vi "LCD_Main Function.vi"(7 "Number of Matches Requested":i32, 8 "error in (no error)":errorcluster, 10 "ROI Descriptor":T3, 11 "Refnum in":T1) -> (0 "error out":errorcluster, 1 "Output value":dbl, 2 "ROI":T2={"Global Rectangle"=[], "Contours"=[{"Contour Type"=0, "ROI Type"=0, "Points"=[27, 55, 147, 27]}]}, 3 "Refnum out":T1)   [LabVIEW 2015]
uses:
  <vilib>/vision/Image Controls.llb/IMAQ Image.ctl
  <vilib>/vision/NI_Vision_Development_Module.lvlib
panel:
  out "Image":T1(plugin-control)
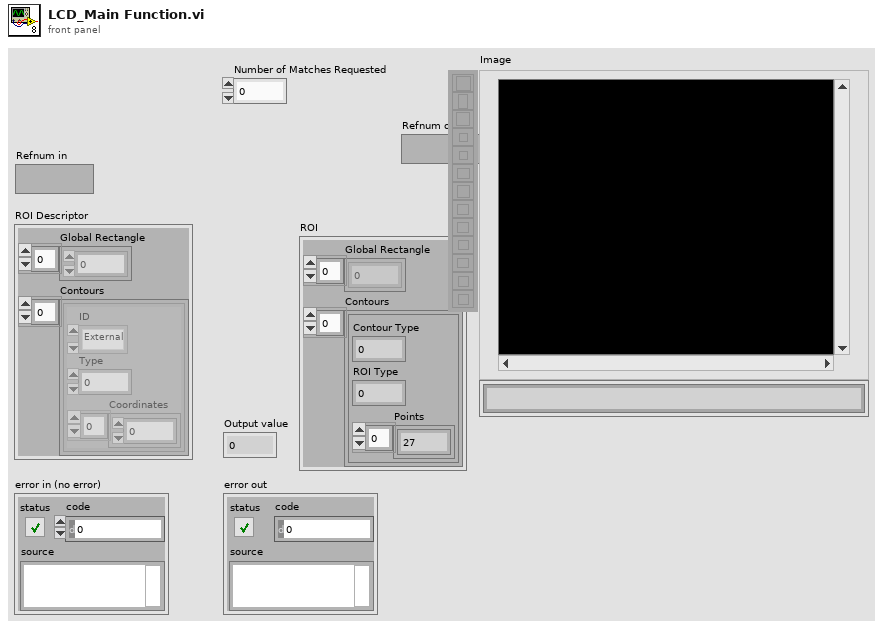
[diagram p1: front panel]
types:
  T1 = typedef "IMAQ Image.ctl" = refnum<image>
  T2 = cluster{"Global Rectangle":i32[], "Contours":cluster{"Contour Type":u32, "ROI Type":u32, "Points":i32[]}[]}
  T3 = cluster{"Global Rectangle":i32[], "Contours":cluster{"ID":enum32{"External", "Internal"}, "Type":u32, "Coordinates":i32[]}[]}
  T4 = cluster{"ID":enum32{"External", "Internal"}, "Type":u32, "Coordinates":i32[]}[]
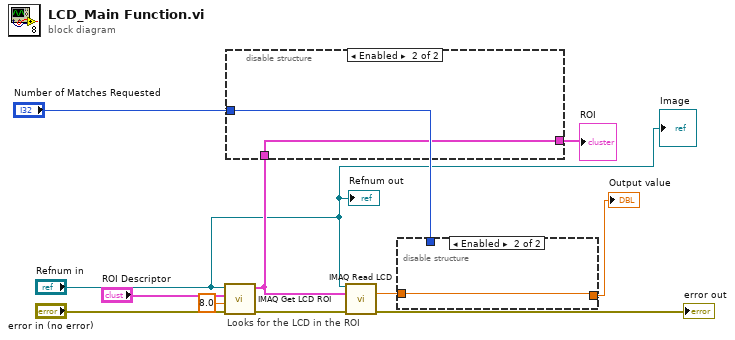
[diagram p0: block diagram]
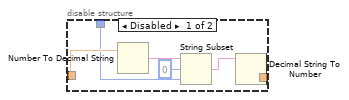
[diagram p2: hidden frame]
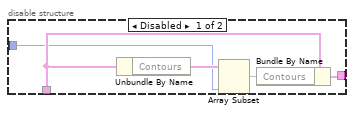
[diagram p3: hidden frame]
diagram:
  # "Looks for the LCD in the ROI"
  n1 = call "IMAQ Get LCD ROI"("error in (no error)"="error in (no error)", "Threshold"=8.0, "ROI Descriptor"="ROI Descriptor", "Image"="Refnum in") -> ("error out"=w9:errorcluster, "ROI Descriptor out"=w7:T3)  [unwired: 6 in]
  n2 = disable-structure shown="Enabled" {
    disable-tunnel: w7 -> [w15 w17]
    disable-tunnel: [w13 w17] -> w6
    disable-tunnel: "Number of Matches Requested" -> [w12 _]
    frame Disabled {
      n3 = Unbundle By Name(w15) -> ("Contours"=w16:T4)
      n4 = Array Subset(array=w16, length=w12) -> (w14:T4)  [unwired: 1 in]
      n5 = Bundle By Name(cluster=w15, "Contours"=w14) -> (w13:T3)
    }
    frame Enabled {
    }
  }
  "ROI" <- w6
  n6 = call "IMAQ Read LCD"("Image"="Refnum in", "ROI Descriptor"=w7, "error in (no error)"=w9) -> ("Output value"=w5:dbl, "error out"=→"error out":errorcluster)  [unwired: 4 in, 7 out]
  n7 = disable-structure shown="Enabled" {
    disable-tunnel: w5 -> [w23 w24]
    disable-tunnel: "Number of Matches Requested" -> [w20 _]
    disable-tunnel: [w18 w24] -> w3
    frame Disabled {
      n8 = Number To Decimal String(number=w23) -> (decimal integer string=w22:string)  [unwired: 1 in]
      n9 = String Subset(string=w22, offset (0)=0, length (rest)=w20) -> (substring=w19:string)
      n10 = Decimal String To Number(string=w19) -> (number=w18:i32)  [unwired: 2 in, 1 out]
    }
    frame Enabled {
    }
  }
  "Output value" <- w3
  "Refnum out" <- "Refnum in"
  "Image" <- "Refnum in"
